vi "ModuleNRSD.vi"(10 "JQMHStartup.lvclass":refnum<class "ModuleStartup.lvclass">, 11 "JQMHCore in":refnum<class "Module.lvclass">) -> ()   [LabVIEW 2024, in "Module.lvclass"]
uses:
  Module.lvclass
  Module.lvclass/Module.ctl
  Startup/ModuleStartup.lvclass
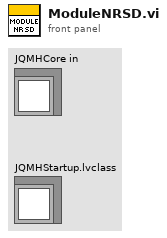
[diagram p1: front panel]
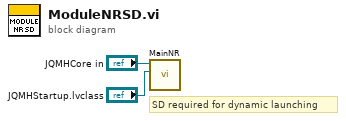
[diagram p0: block diagram]
diagram:
  # "SD required for dynamic launching"
  n1 = call-dynamic "MainNR.vi"("JQMHStartup.lvclass"="JQMHStartup.lvclass", "JQMHCore in"="JQMHCore in") -> ()  [unwired: 10 in]
